vi "Load.vi"(8 "error in (no error)":errorcluster, 9 "Config path":path caption="Configuration file path (leave empty to load default path)", 10 "VI path":path caption="VI path to load default controls") -> (0 "error out":errorcluster, 2 "Configuration file path (*.ini)":path, 3 "Default contorls manipulator out":refnum<class "Default contorls manipulator.lvclass">)   [LabVIEW 2020, in "Default contorls manipulator.lvclass"]
doc: "Simply wire <b>Current VI's Path</b> to the input to load previously saved configuration file (default path: .data/*_config.ini). If the configuration file is not existed, this VI create one.\n\nThe configuration file is in <b>ini</b> format and save to path <b>./data/[Current VI's file name]+_config.ini</b>. Users can overwrite the default path by assigning a new <b>Configuration file path</b>.\n\nNote that the LOAD operation is typically run in the early stage of a program."
uses:
  Default contorls manipulator.lvclass
  Default contorls manipulator.lvclass/Default contorls manipulator.ctl
  Save-Load-Defaults.lvlib/Save-Load-Defaults.lvlib
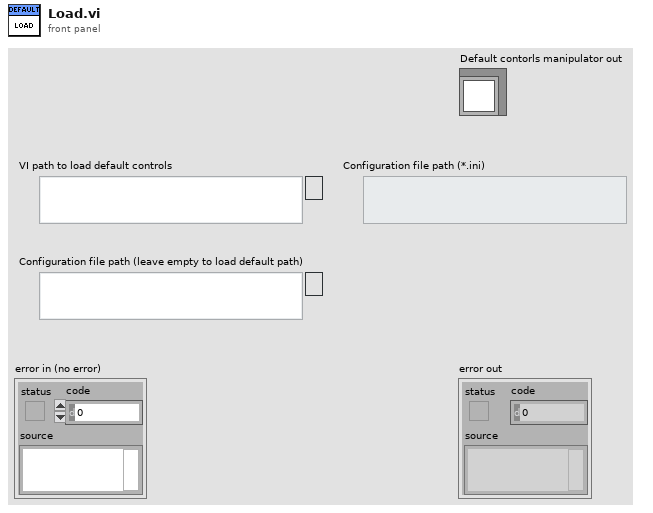
[diagram p1: front panel]
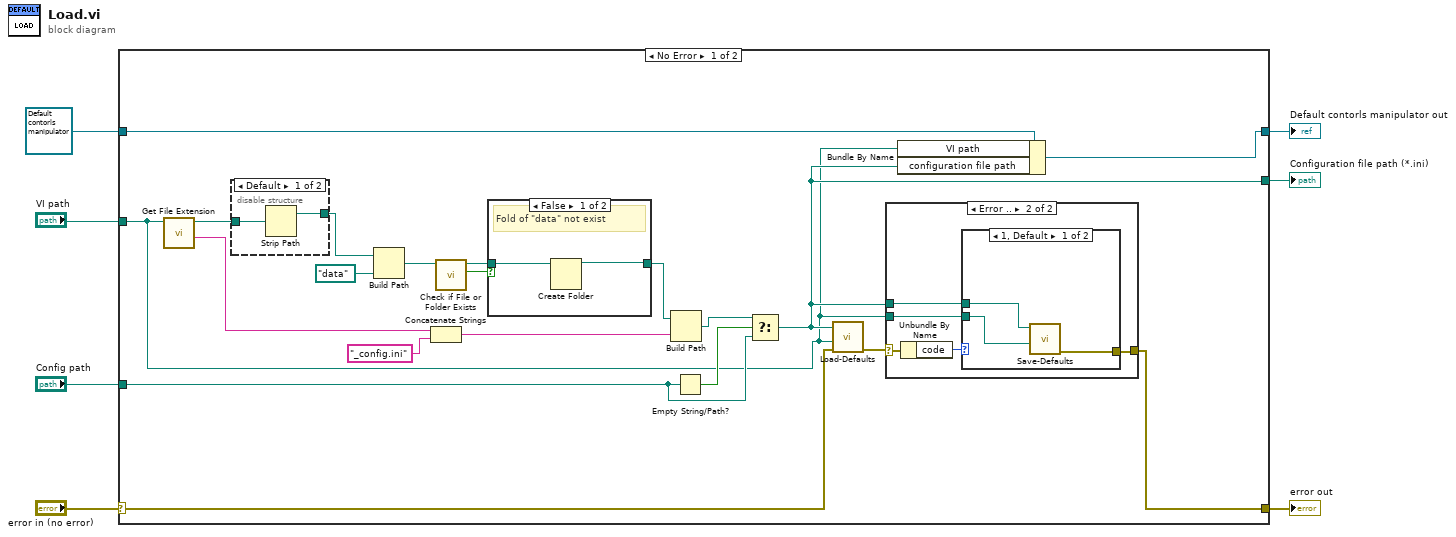
[diagram p0: block diagram]
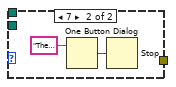
[diagram p3: hidden frame]
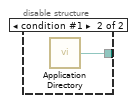
[diagram p4: hidden frame]
diagram:
  n1 = case shown="No Error" "error in (no error)" {
    selector: "error in (no error)" -> [w17 w46]
    tunnel: [w15 w46] -> w6
    tunnel: refnum<class "Default contorls manipulator.lvclass"> refnum ("Default contorls manipulator.lvclass") -> [w11 w45]
    tunnel: [w10 w45] -> w4
    tunnel: "VI path" -> [w8 _]
    tunnel: "Config path" -> [w12 _]
    tunnel: [w9 _] -> w1
    frame No Error {
      n2 = call <vilib>:"Get File Extension.vi"("file"=w8) -> ("filename without extension"=w27:string, "dup file"=w19:path)  [unwired: 6 in, 3 out]
      n3 = disable-structure shown="Default" {
        disable-tunnel: w19 -> [w40 _]
        disable-tunnel: [w39 w41] -> w18
        frame condition #0 (active) {
          n4 = Strip Path(path=w40) -> (stripped path=w39:path)  [unwired: 1 out]
        }
        frame condition #1 {
          n5 = call <vilib>:"Application Directory.vi"() -> ("Application Directory"=w41:path)
        }
      }
      n6 = Build Path(base path=w18, name or relative path=path "data") -> (appended path=w23:path)
      n7 = Concatenate Strings(w27, "_config.ini" ("string")) -> (w24:string)
      n8 = call <vilib>:"Check if File or Folder Exists.vi"("path"=w23) -> ("file or folder exists?"=w22:bool, "dup path"=w21:path)  [unwired: 8 in, 1 out]
      n9 = case shown="False" w22 {
        tunnel: w21 -> [w43 w44]
        tunnel: [w42 w44] -> w20
        frame False {
          # "Fold of \"data\" not exist"
          n10 = Create Folder(path (use dialog)=w43) -> (created path=w42:path)  [unwired: 2 in, 2 out]
        }
        frame True {
          # "Folder \"data\" existed"
        }
      }
      n11 = Build Path(base path=w20, name or relative path=w24) -> (appended path=w14:path)
      n12 = Empty String/Path?(string/path=w12) -> (empty?=w13:bool)
      n13 = Select(t=w14, s=w13, f=w12) -> (s? t:f=w9:path)
      n14 = call "Load-Defaults.vi"("error in (no error)"=w17, "VI path"=w8, "configuration file path"=w9) -> ("error out"=w16:errorcluster)  [unwired: 8 in]
      n15 = case shown="Error .." w16 {
        selector: w16 -> [w28 w33]
        tunnel: [w28 w31] -> w15
        tunnel: w9 -> [_ w30]
        tunnel: w8 -> [_ w29]
        frame No Error {
        }
        frame Error {
          n16 = Unbundle By Name(w33) -> ("code"=w32:i32)
          n17 = case shown="1, Default" w32 {
            tunnel: [w36 _] -> w31
            tunnel: w30 -> [w35 _]
            tunnel: w29 -> [w34 _]
            frame 1, Default {
              n18 = call "Save-Defaults.vi"("VI path"=w34, "configuration file path"=w35) -> ("error out"=w36:errorcluster)  [unwired: 9 in]
            }
            frame 7 {
              n19 = One Button Dialog(message="The path to INI file or INI format is invalid.\n\nProgram will be quit.\n\n(Error 7)") -> (true=w37:bool)  [unwired: 1 in]
              n20 = Stop(stop? (T)=w37) -> ()
            }
          }
        }
      }
      n21 = Bundle By Name(cluster=w11, "VI path"=w8, "configuration file path"=w9) -> (w10:refnum<class "Default contorls manipulator.lvclass">)
    }
    frame Error {
    }
  }
  "error out" <- w6
  "Default contorls manipulator out" <- w4
  "Configuration file path (*.ini)" <- w1
